vi "OutputDirectory.vi"() -> ()   [LabVIEW 2013]
panel:
  out "Output Directory":path
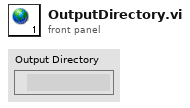
[diagram p1: front panel]
diagram:
